vi "CAN_Filter.vi"(0 "NTC":T1, 1 "VCELL":T1, 2 "SOC SOH":T1, 3 "Current":T1, 4 "Error1":T1) -> (7 "Tableau":dbl[](array[numeric]))   [LabVIEW 2020]
panel:
  out "x/y":dbl
  in  "Current 2":u8[](array[numeric])
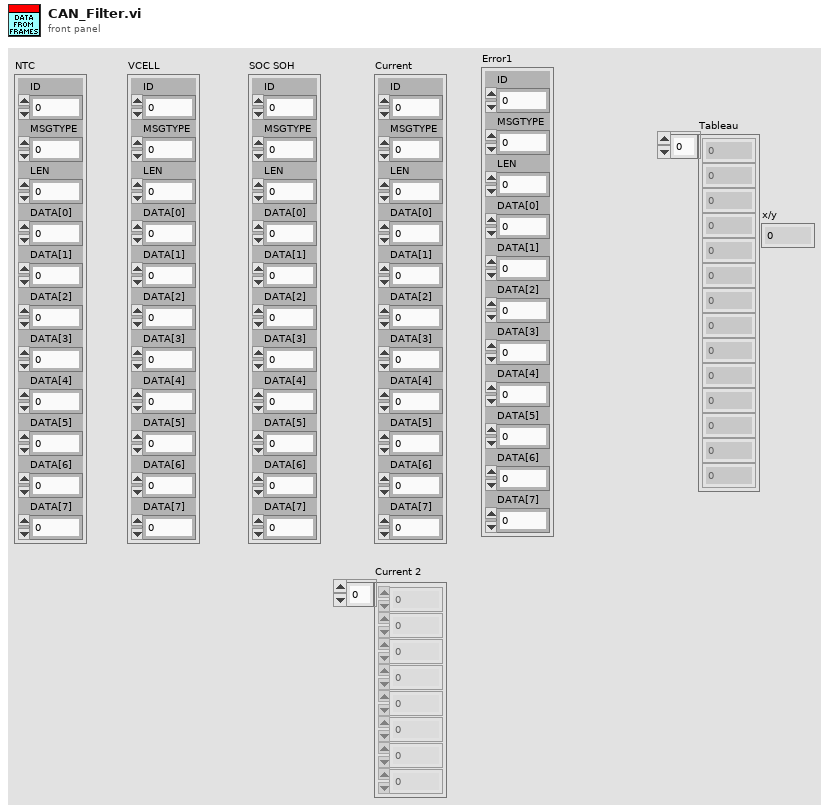
[diagram p1: front panel]
types:
  T1 = cluster{"ID":u32, "MSGTYPE":u8, "LEN":u8, "DATA[0]":u8, "DATA[1]":u8, "DATA[2]":u8, "DATA[3]":u8, "DATA[4]":u8, "DATA[5]":u8, "DATA[6]":u8, "DATA[7]":u8}
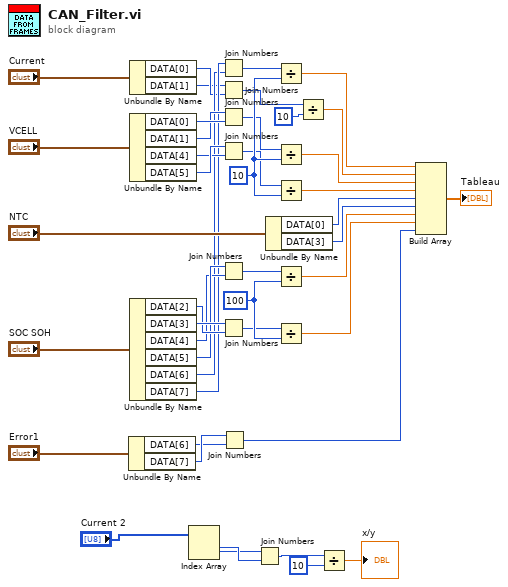
[diagram p0: block diagram]
diagram:
  w40 = u16 100 ("y")
  w39 = u16 10 ("y")
  n1 = Unbundle By Name("Error1") -> ("DATA[6]"=w8:u8, "DATA[7]"=w9:u8)
  n2 = Unbundle By Name("Current") -> ("DATA[0]"=w21:u8, "DATA[1]"=w20:u8)
  n3 = Unbundle By Name("VCELL") -> ("DATA[0]"=w36:u8, "DATA[1]"=w35:u8, "DATA[4]"=w32:u8, "DATA[5]"=w33:u8)
  n4 = Unbundle By Name("SOC SOH") -> ("DATA[2]"=w29:u8, "DATA[3]"=w30:u8, "DATA[4]"=w26:u8, "DATA[5]"=w27:u8, "DATA[6]"=w23:u8, "DATA[7]"=w24:u8)
  n5 = Index Array(array="Current 2") -> (element #1=w5:u8, element #2=w4:u8)  [unwired: 2 in]
  n6 = Join Numbers(hi=w24, lo=w23) -> ((hi.lo)=w22:u16)
  n7 = Join Numbers(hi=w20, lo=w21) -> ((hi.lo)=w19:u16)
  n8 = Join Numbers(hi=w35, lo=w36) -> ((hi.lo)=w34:u16)
  n9 = Join Numbers(hi=w33, lo=w32) -> ((hi.lo)=w31:u16)
  n10 = Join Numbers(hi=w27, lo=w26) -> ((hi.lo)=w25:u16)
  n11 = Join Numbers(hi=w30, lo=w29) -> ((hi.lo)=w28:u16)
  n12 = Join Numbers(hi=w9, lo=w8) -> ((hi.lo)=w7:u16)
  n13 = Join Numbers(hi=w4, lo=w5) -> ((hi.lo)=w3:u16)
  n14 = Unbundle By Name("NTC") -> ("DATA[0]"=w14:u8, "DATA[3]"=w13:u8)
  n15 = Divide(x=w22, y=w39) -> (x/y=w18:dbl)
  n16 = Divide(x=w34, y=w39) -> (x/y=w16:dbl)
  n17 = Divide(x=w31, y=w39) -> (x/y=w15:dbl)
  n18 = Divide(x=w25, y=w40) -> (x/y=w11:dbl)
  n19 = Divide(x=w28, y=w40) -> (x/y=w44:dbl)
  n20 = Divide(x=w19, y=u16 10) -> (x/y=w17:dbl)
  n21 = Divide(x=w3, y=u16 10) -> (x/y=→"x/y":dbl)
  n22 = Build Array(w18, w17, w16, w15, w14, w13, w11, w44, w7) -> (→"Tableau":dbl[])
